vi "Update Navigation.vi"(8 "error in (no error)":errorcluster, 9 "Data":variant, 10 "Name":string, 11 "Ctl Target":T1) -> (0 "error out":errorcluster)   [LabVIEW 2020, in "Navigation.lvlib"]
doc: "<b>Note</b>: This VI was renamed by the DQMH Rename Event utility. Make sure the VI Description is updated to reflect the new event name, then delete this comment.\n\nSend information for updating the Sidebar to some state.\n____\nHAMPEL SOFTWARE ENGINEERING v2.6.0 (2023-12-19 10:54)"
uses:
  Navigation.lvlib
  Sub-VIs/Ctl Target.ctl
  Update Navigation Argument--cluster.ctl
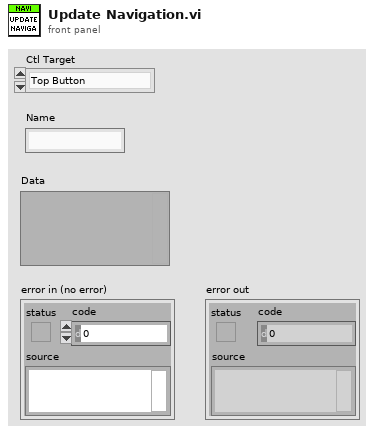
[diagram p1: front panel]
types:
  T1 = typedef "Navigation.lvlib/Ctl Target.ctl" = enum16{"Top Button", "Sub ListBox"}
  T2 = typedef "Navigation.lvlib/Update Navigation Argument--cluster.ctl" = cluster{"Ctl Target":T1, "Name":string, "Data":variant}
  T3 = typedef "Navigation.lvlib/Request Events--cluster.ctl" = cluster{"Stop Module":refnum<user-event>, "Show Panel":refnum<user-event>, "Hide Panel":refnum<user-event>, "Get Module Execution Status":refnum<user-event>, "Show Diagram":refnum<user-event>, "Prepare":refnum<user-event>, "Update Navigation":refnum<user-event>, "Configure":refnum<user-event>, "Select Listbox Element":refnum<user-event>, "Set Visibility":refnum<user-event>, "Set Disabled State":refnum<user-event>}
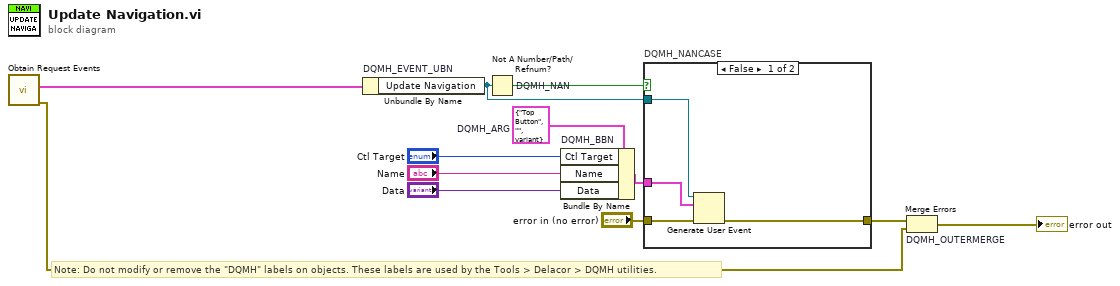
[diagram p0: block diagram]
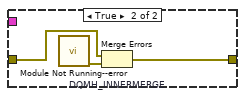
[diagram p2: hidden frame]
diagram:
  w6 = T2 {"Ctl Target"=enum."Top Button", "Name"="", "Data"=variant}  # DQMH_ARG
  # "Note: Do not modify or remove the \"DQMH\" labels on objects. These labels are used by the Tools > Delacor > DQMH utilities."
  n1 = call "Obtain Request Events.vi"() -> ("error out"=w3:errorcluster, "Navigation Request Events"=w2:T3)  [unwired: 10 in]
  n2 = Unbundle By Name "DQMH_EVENT_UBN"(w2) -> ("Update Navigation"=w8:refnum<user-event>)
  n3 = Not A Number/Path/Refnum? "DQMH_NAN"(number/path/refnum=w8) -> (NaN/Path/Refnum?=w9:bool)
  n4 = Bundle By Name "DQMH_BBN"(cluster=w6, "Ctl Target"="Ctl Target", "Name"="Name", "Data"="Data") -> (w10:T2)
  n5 = case "DQMH_NANCASE" shown="False" w9 {
    tunnel: "error in (no error)" -> [w16 w19]
    tunnel: [w15 w18] -> w7
    tunnel: w8 -> [w14 _]
    tunnel: w10 -> [w13 _]
    frame False {
      n6 = Generate User Event(user event=w14, event data cluster=w13, error in=w16) -> (error out=w15:errorcluster)  [unwired: 1 in, 1 out]
    }
    frame True {
      n7 = call "Module Not Running--error.vi"() -> ("error out"=w17:errorcluster)  [unwired: 11 in]
      n8 = Merge Errors "DQMH_INNERMERGE"(w19, w17) -> (w18:errorcluster)
    }
  }
  n9 = Merge Errors "DQMH_OUTERMERGE"(w7, w3) -> (→"error out":errorcluster)
